vi "Actor Template-Core_Process.vi"(0 "FTW Actor Instance Configuration":string="{\n  \"Identity\": \"ActorName\",\n  \"InboxAddress\": \"inproc://*\",\n  \"LoggerAddress\": \"\",\n  \"My Data\": false,\n  \"Publisher URI\": \"inproc://*\",\n  \"Subscriber URIs\": \"\",\n  \"Refresh Period\": 2\n}", 11 "ErrorIn":errorcluster) -> (15 "Error":errorcluster)   [LabVIEW 2015, in "Actor Template-Core.lvclass"]
uses:
  Actor Template-Core.lvclass
  Actor Template-Core.lvclass/Actor Template-Core.ctl
  source/actor/Instance/FTW-ActorInstance.lvclass/FTW-ActorInstance.ctl
  source/actor/JobSequencer/FTW-SEQ-Current.vi
  source/actor/Message/Base/FTW-Message.lvclass
  source/actor/Connector/FTW-ActorConnector.lvclass
  source/actor/Instance/FTW-ActorInstance.lvclass
  source/actor/Message/Request/FTW-Message-IncomingRequest.lvclass
  source/actor/Publisher/FTW-Publisher.lvclass
  source/actor/Subscriber/FTW-Subscriber.lvclass
panel:
  # "#TODO\nhide controls for a GUI"
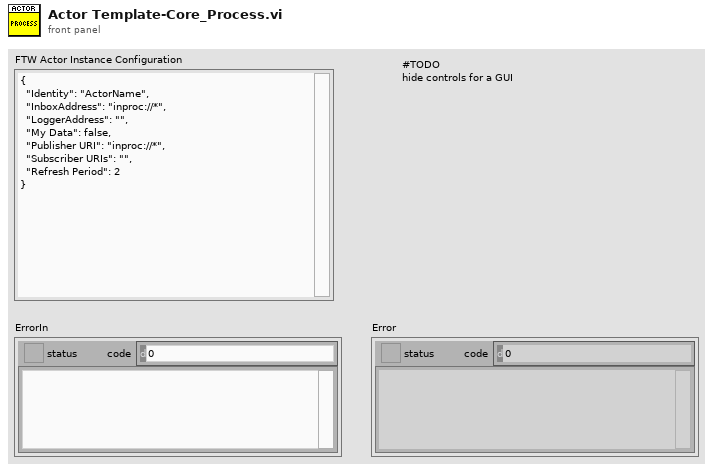
[diagram p1: front panel]
types:
  T1 = cluster{"Incoming Requests":refnum<event-registration>, "Local Messages":refnum<event-registration>, "Subscriber Registration":refnum<event-registration>}
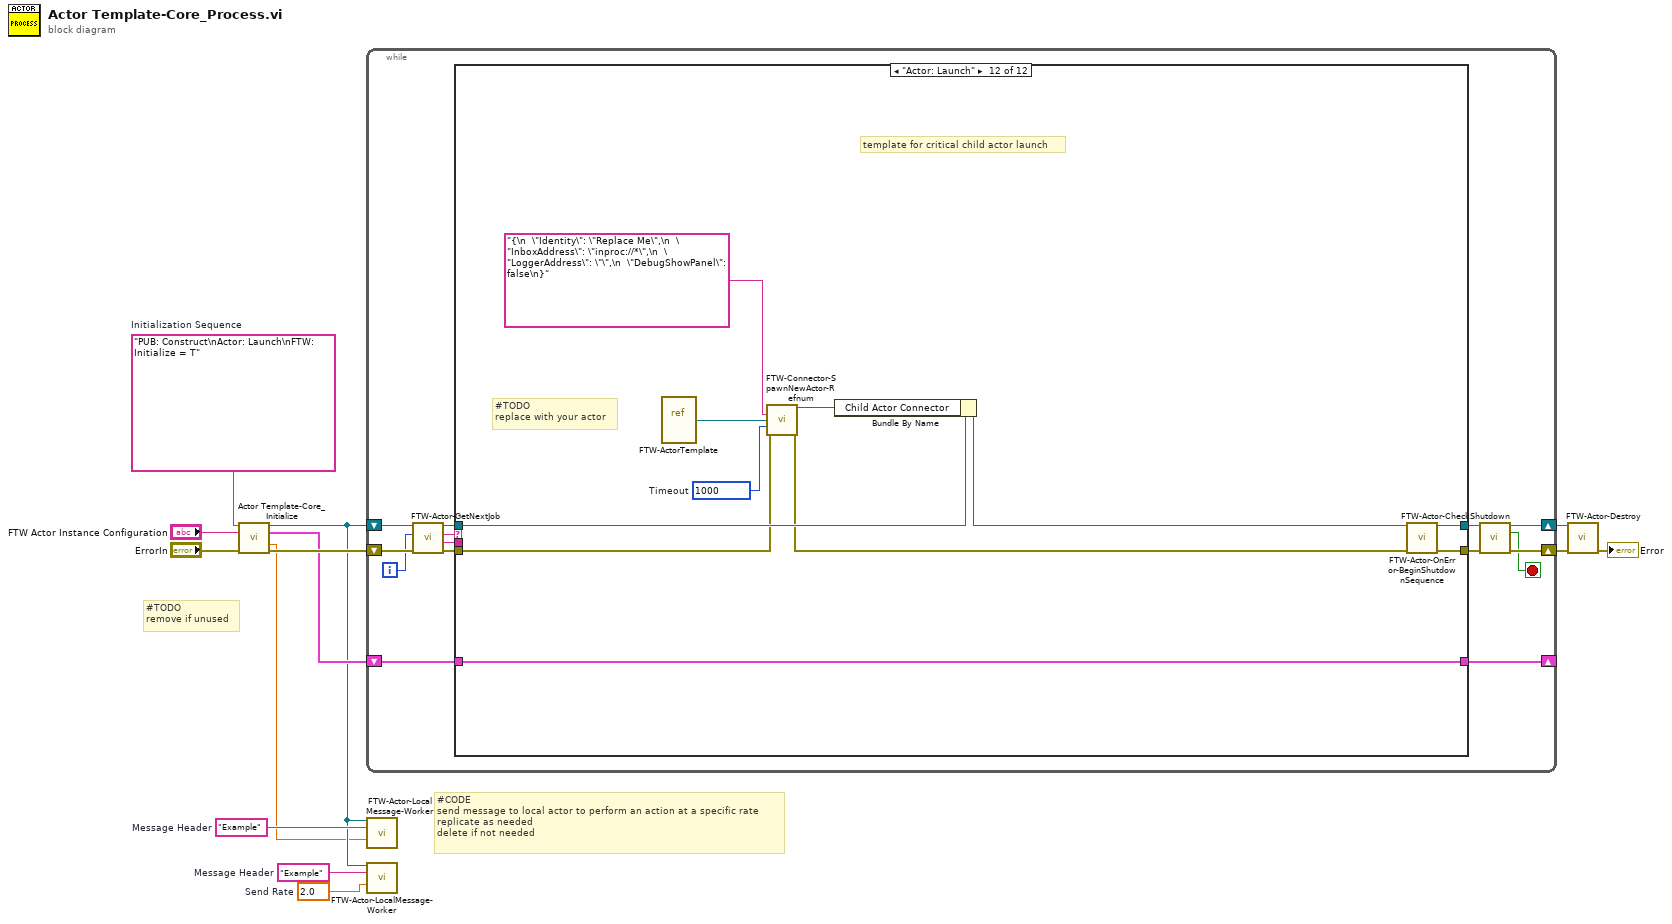
[diagram p0: block diagram]
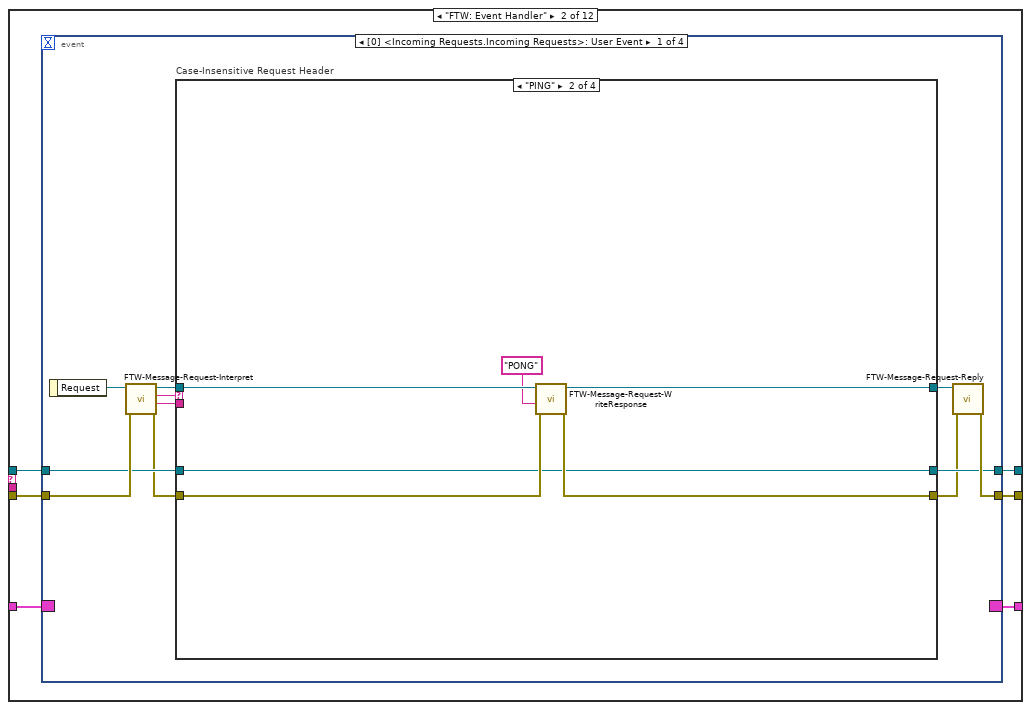
[diagram p3: hidden frame]
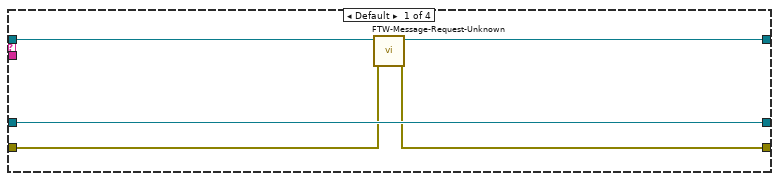
[diagram p4: hidden frame]
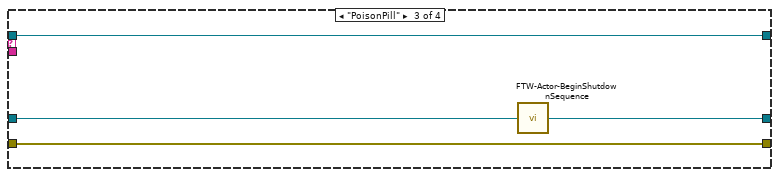
[diagram p5: hidden frame]
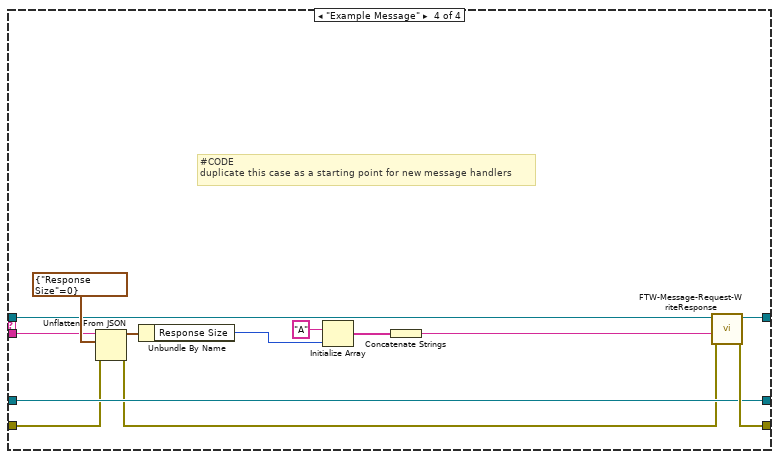
[diagram p6: hidden frame]
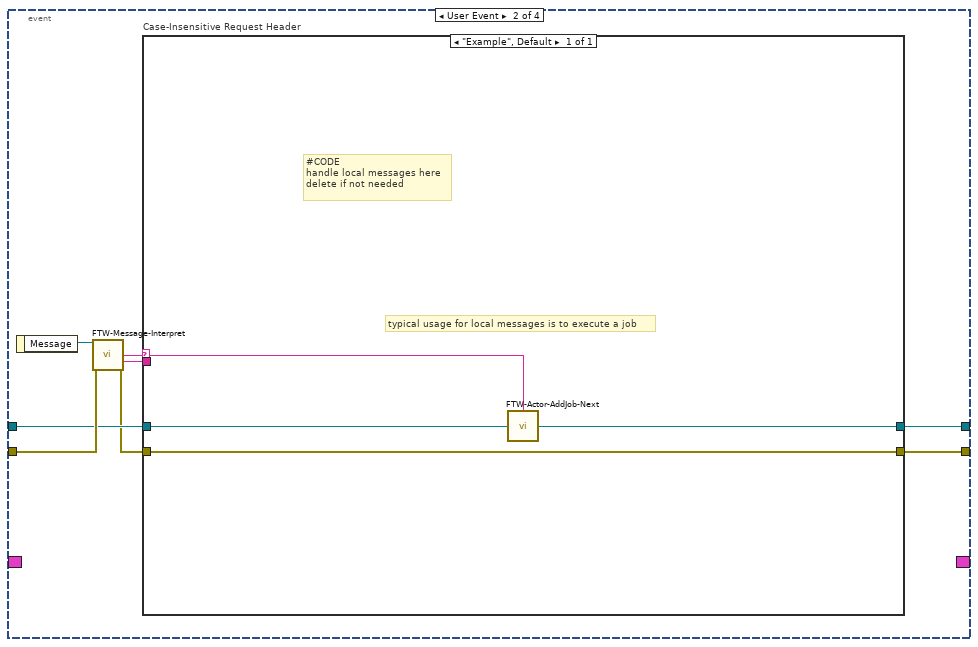
[diagram p7: hidden frame]
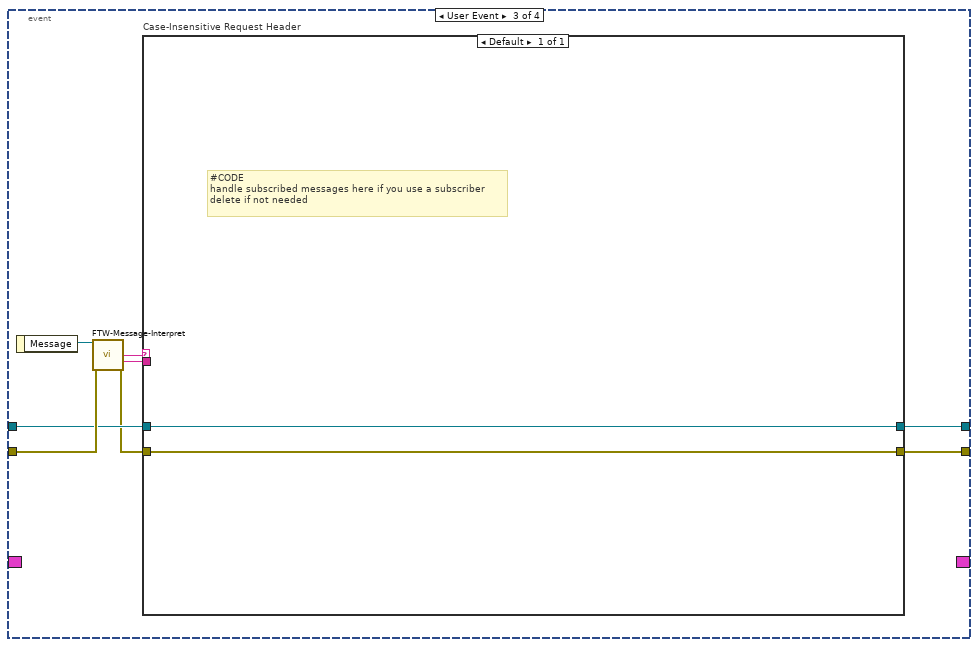
[diagram p8: hidden frame]
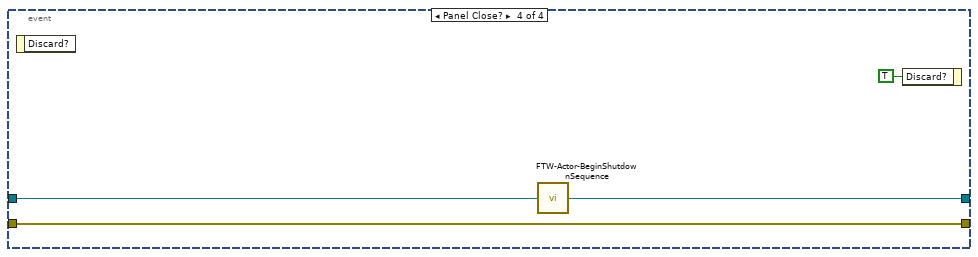
[diagram p9: hidden frame]
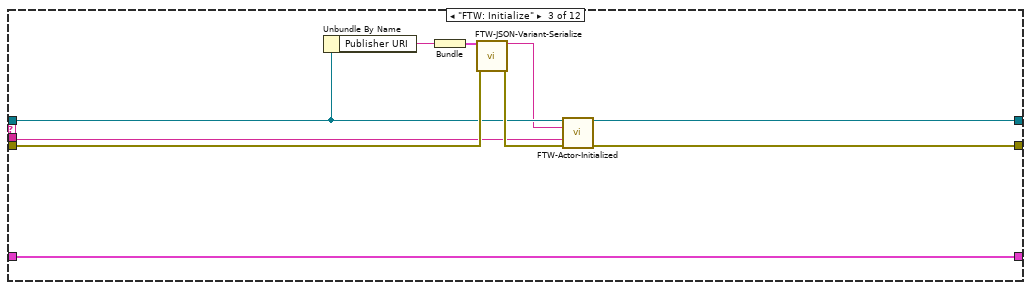
[diagram p10: hidden frame]
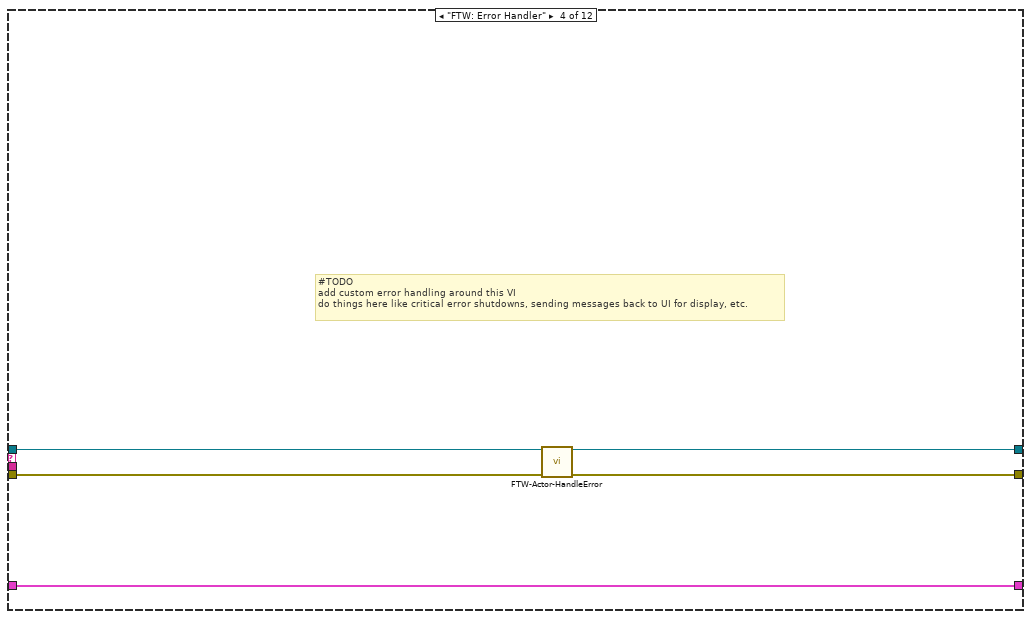
[diagram p11: hidden frame]
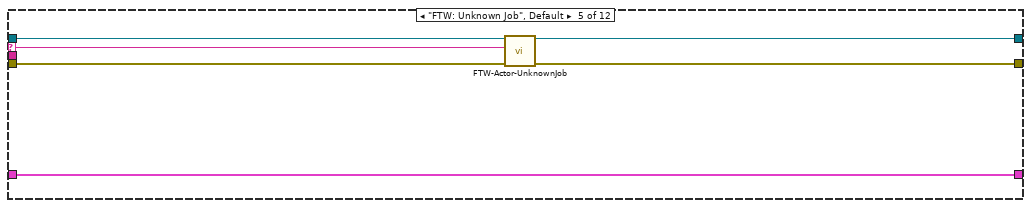
[diagram p12: hidden frame]
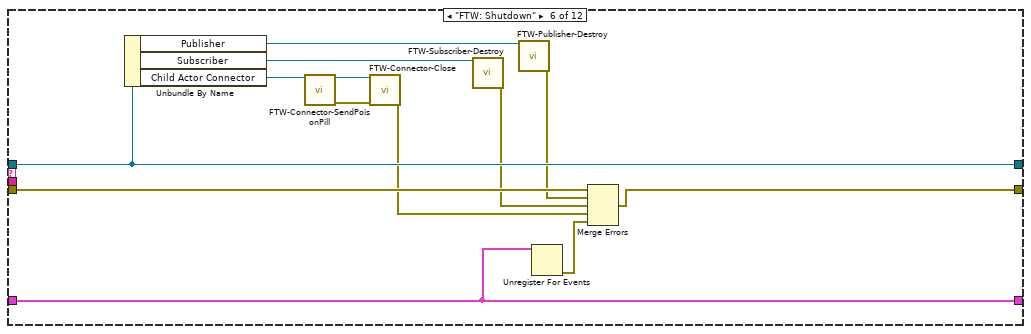
[diagram p13: hidden frame]
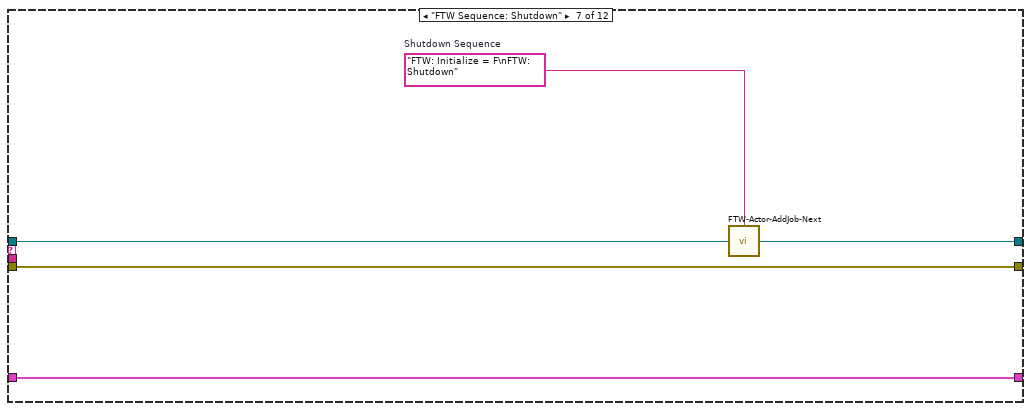
[diagram p14: hidden frame]
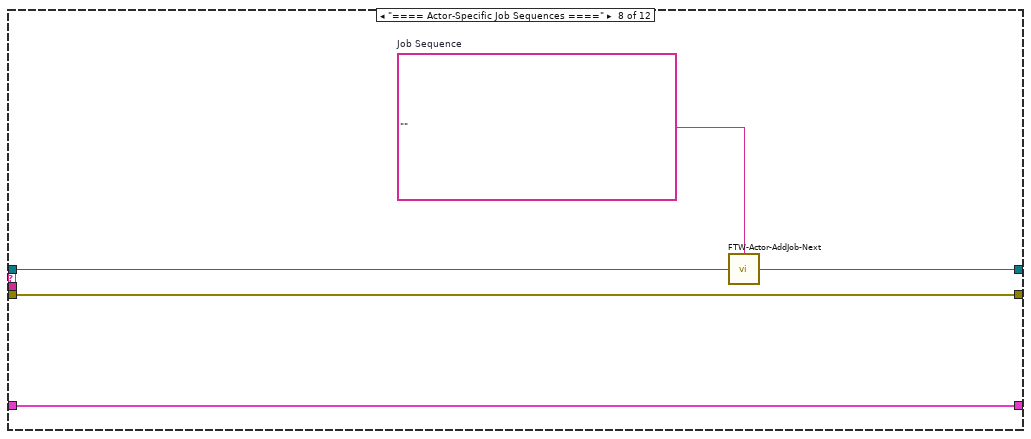
[diagram p15: hidden frame]
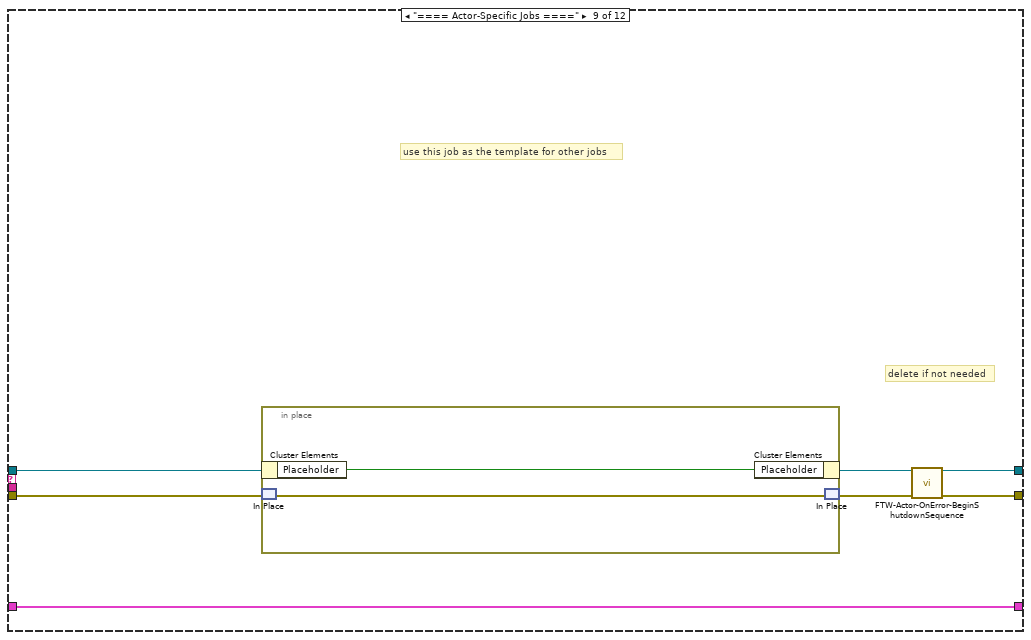
[diagram p16: hidden frame]
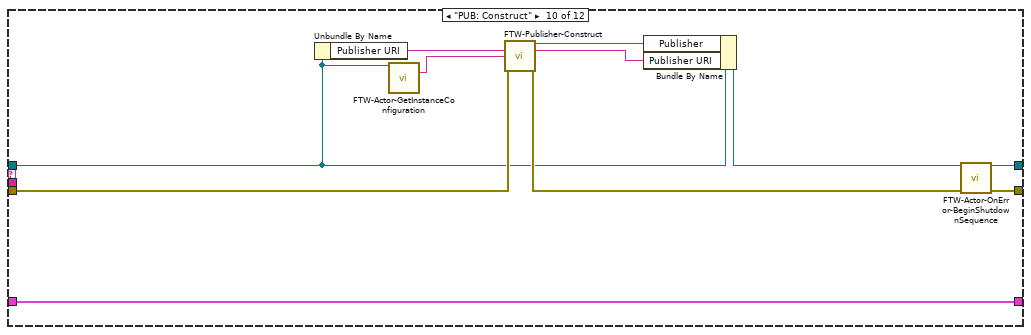
[diagram p17: hidden frame]
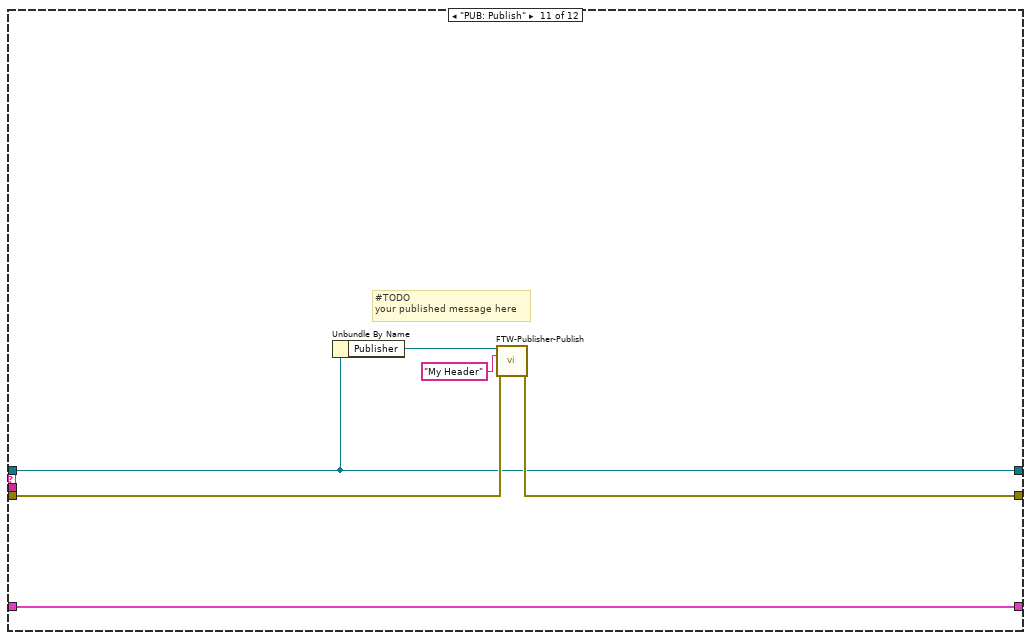
[diagram p18: hidden frame]
diagram:
  w4 = 2.0  # Send Rate
  w3 = "Example"  # Message Header
  w5 = "Example"  # Message Header
  w9 = "PUB: Construct\nActor: Launch\nFTW: Initialize = T"  # Initialization Sequence
  # "#CODE\nsend message to local actor to perform an action at a specific rate\nreplicate as needed\ndelete if not needed"
  # "#TODO\nremove if unused"
  n1 = call "Actor Template-Core_Initialize.vi"("Initialization Sequence"=w9, "FTW Actor Instance Configuration"="FTW Actor Instance Configuration", "error in (no error)"="ErrorIn") -> ("Actor Template-Core out"=w2:refnum<class "Actor Template-Core.lvclass">, "Event Refnums"=w6:T1, "Refresh Period"=w1:dbl, "error out"=w10:errorcluster)  [unwired: 9 in]
  n2 = while {
    shift-right: [w17] -> w12
    shift-left: w10 -> [w24]
    shift-right: [w14] -> _
    shift-left: w6 -> [w27]
    shift-right: [w19] -> w13
    shift-left: w2 -> [w26]
    i -> [w15]
    stop <- w16 stop-if-true
    n3 = call "FTW-Actor-GetNextJob.vi"("error in"=w24, "Jobs Performed"=w15, "FTW Actor Instance"=w26) -> ("error out"=w23:errorcluster, "Job Data"=w21:string, "Job Name"=w22:string, "FTW Actor Instance out"=w25:refnum<class "Actor Template-Core.lvclass">)  [unwired: 5 in]
    n4 = case shown="\"Actor: Launch\"" w22 {
      selector: w22 -> [_ _ _ _ w117 _ _ _ _ _ _ _]
      tunnel: [w29 w36 w107 w112 w120 w134 w139 w144 w148 w161 w169 w181] -> w18
      tunnel: w23 -> [w29 w35 w111 w114 w121 w135 w139 w144 w151 w163 w170 w175]
      tunnel: w27 -> [w30 w31 w109 w116 w122 w132 w140 w145 w152 w165 w171 w182]
      tunnel: [w30 w34 w109 w116 w122 w132 w140 w145 w152 w165 w171 w182] -> w14
      tunnel: w21 -> [_ _ w104 _ _ _ _ _ _ _ _ _]
      tunnel: [w28 w33 w108 w113 w118 w131 w137 w142 w146 w159 w168 w180] -> w20
      tunnel: w25 -> [w28 w32 w106 w115 w119 w131 w138 w143 w149 w156 w168 w179]
      frame "==== Featherweight Framework Jobs ====" {
      }
      frame "FTW: Event Handler" {
        n5 = event shown="[0] <Incoming Requests.Incoming Requests>: User Event" {
          selector: w31 -> [_ _ _ _]
          dyn-events: [_ _ _ _] -> w34
          timeout: _ -> [_ _ _ _]
          tunnel: [w46 w78 w90 w100] -> w36
          tunnel: w35 -> [w45 w82 w94 w100]
          tunnel: [w40 w79 w91 w98] -> w33
          tunnel: w32 -> [w44 w81 w93 w99]
          event User Event {
            n6 = event-data() -> ("Request"=w47:refnum<class "FTW-Message-IncomingRequest.lvclass">)  [unwired: 1 in]
            n7 = call "FTW-Message-Request-Interpret.vi"("error in"=w45, "FTW Incoming Request"=w47) -> ("error out"=w43:errorcluster, "Request Body"=w37:string, "Request Header"=w41:string, "FTW Incoming Request out"=w42:refnum<class "FTW-Message-IncomingRequest.lvclass">)  [unwired: 6 in]
            n8 = case "Case-Insensitive Request Header" shown="\"PING\"" w41 {
              tunnel: [w50 w56 w61 w75] -> w39
              tunnel: w43 -> [w51 w57 w61 w64]
              tunnel: [w52 w55 w62 w73] -> w40
              tunnel: w44 -> [w52 w55 w60 w73]
              tunnel: w42 -> [w49 w58 w59 w65]
              tunnel: [w48 w54 w59 w74] -> w38
              tunnel: w37 -> [_ _ _ w63]
              frame Default {
                n9 = call "FTW-Message-Request-Unknown.vi"("error in"=w51, "FTW Incoming Request"=w49) -> ("error out"=w50:errorcluster, "FTW Incoming Request Out"=w48:refnum<class "FTW-Message-IncomingRequest.lvclass">)  [unwired: 8 in]
              }
              frame "PING" {
                n10 = call "FTW-Message-Request-WriteResponse.vi"("error in"=w57, "Response Body"="PONG" ("Response Header"), "FTW Incoming Request"=w58) -> ("error out"=w56:errorcluster, "FTW Incoming Request out"=w54:refnum<class "FTW-Message-IncomingRequest.lvclass">)  [unwired: 7 in]
              }
              frame "PoisonPill" {
                n11 = call "FTW-Actor-BeginShutdownSequence.vi"("FTW Actor Instance"=w60) -> ("FTW Actor Instance out"=w62:refnum<class "Actor Template-Core.lvclass">)  [unwired: 3 in]
              }
              frame "Example Message" {
                # "#CODE\nduplicate this case as a starting point for new message handlers"
                n12 = Unflatten From JSON(JSON string=w63, type and defaults=cluster{"Response Size":i32} {"Response Size"=0}, error in (no error)=w64) -> (value=w70:cluster{"Response Size":i32}, error out=w72:errorcluster)  [unwired: 4 in]
                n13 = Unbundle By Name(w70) -> ("Response Size"=w69:i32)
                n14 = Initialize Array("A", w69) -> (w67:string[])
                n15 = Concatenate Strings(w67) -> (w66:string)
                n16 = call "FTW-Message-Request-WriteResponse.vi"("error in"=w72, "Response Body"=w66, "FTW Incoming Request"=w65) -> ("error out"=w75:errorcluster, "FTW Incoming Request out"=w74:refnum<class "FTW-Message-IncomingRequest.lvclass">)  [unwired: 7 in]
              }
            }
            n17 = call "FTW-Message-Request-Reply.vi"("FTW: Reply Error"=w39, "FTW Incoming Request"=w38) -> ("error out"=w46:errorcluster)  [unwired: 8 in, 1 out]
          }
          event User Event {
            n18 = event-data() -> ("Message"=w83:refnum<class "FTW-Message.lvclass">)  [unwired: 1 in]
            n19 = call-dynamic "FTW-Message-Interpret.vi"("FTW Message"=w83, "error in"=w82) -> ("Message Header"=w77:string, "Message Body"=w76:string, "error out"=w80:errorcluster)  [unwired: 9 in, 2 out]
            n20 = case "Case-Insensitive Request Header" shown="\"Example\", Default" w77 {
              selector: w77 -> [w84]
              tunnel: [w86] -> w78
              tunnel: w80 -> [w86]
              tunnel: [w85] -> w79
              tunnel: w81 -> [w87]
              tunnel: w76 -> [_]
              frame "Example", Default {
                # "#CODE\nhandle local messages here\ndelete if not needed"
                # "typical usage for local messages is to execute a job"
                n21 = call "FTW-Actor-AddJob-Next.vi"("Add Next in Job Queue"=w84, "FTW Actor Instance"=w87) -> ("FTW Actor Instance out"=w85:refnum<class "Actor Template-Core.lvclass">)  [unwired: 2 in]
              }
            }
          }
          event User Event {
            n22 = event-data() -> ("Message"=w95:refnum<class "FTW-Message.lvclass">)  [unwired: 1 in]
            n23 = call-dynamic "FTW-Message-Interpret.vi"("FTW Message"=w95, "error in"=w94) -> ("Message Header"=w89:string, "Message Body"=w88:string, "error out"=w92:errorcluster)  [unwired: 9 in, 2 out]
            n24 = case "Case-Insensitive Request Header" shown="Default" w89 {
              tunnel: [w96] -> w90
              tunnel: w92 -> [w96]
              tunnel: [w97] -> w91
              tunnel: w93 -> [w97]
              tunnel: w88 -> [_]
              frame Default {
                # "#CODE\nhandle subscribed messages here if you use a subscriber\ndelete if not needed"
              }
            }
          }
          event Panel Close? {
            n25 = event-data() -> ()  [unwired: 1 in, 1 out]
            n26 = call "FTW-Actor-BeginShutdownSequence.vi"("FTW Actor Instance"=w99) -> ("FTW Actor Instance out"=w98:refnum<class "Actor Template-Core.lvclass">)  [unwired: 3 in]
            n27 = event-data("Discard?"=TRUE) -> ()  [unwired: 1 in, 1 out]
          }
        }
      }
      frame "FTW: Initialize" {
        n28 = Unbundle By Name(w106) -> ("Publisher URI"=w105:string)
        n29 = Bundle("Publisher URI"=w105) -> (w103:cluster{"Publisher URI":string})  [unwired: 1 in]
        n30 = call "FTW-JSON-Variant-Serialize.vi"("Variant"=w103, "error in"=w111) -> ("JSON String"=w102:string, "error out"=w110:errorcluster)  [unwired: 12 in]
        n31 = call-dynamic "FTW-Actor-Initialized.vi"("FTW Actor Instance"=w106, "Initialized Response"=w102, "Positive Init?"=w104, "error in"=w110) -> ("FTW Actor Instance out"=w108:refnum<class "Actor Template-Core.lvclass">, "error out"=w107:errorcluster)  [unwired: 10 in]
      }
      frame "FTW: Error Handler" {
        # "#TODO\nadd custom error handling around this VI\ndo things here like critical error shutdowns, sending messages back to UI for display, etc."
        n32 = call-dynamic "FTW-Actor-HandleError.vi"("FTW Actor Instance"=w115, "error in"=w114) -> ("FTW Actor Instance out"=w113:refnum<class "Actor Template-Core.lvclass">, "error out"=w112:errorcluster)  [unwired: 10 in, 2 out]
      }
      frame "FTW: Unknown Job", Default {
        n33 = call-dynamic "FTW-Actor-UnknownJob.vi"("FTW Actor Instance"=w119, "Unknown Job"=w117, "error in"=w121) -> ("FTW Actor Instance out"=w118:refnum<class "Actor Template-Core.lvclass">, "error out"=w120:errorcluster)  [unwired: 11 in]
      }
      frame "FTW: Shutdown" {
        n34 = Unbundle By Name(w131) -> ("Publisher"=w130:refnum<class "FTW-Publisher.lvclass">, "Subscriber"=w128:refnum<class "FTW-Subscriber.lvclass">, "Child Actor Connector"=w126:refnum<class "FTW-ActorConnector.lvclass">)
        n35 = call-dynamic "FTW-Connector-SendPoisonPill.vi"("FTW Actor Connector"=w126) -> ("FTW Actor Connector out"=w125:refnum<class "FTW-ActorConnector.lvclass">, "error out"=w124:errorcluster)  [unwired: 9 in, 4 out]
        n36 = call-dynamic "FTW-Connector-Close.vi"("FTW Actor Connector"=w125, "error in"=w124) -> ("error out"=w123:errorcluster)  [unwired: 13 in]
        n37 = call "FTW-Subscriber-Destroy.vi"("FTW-Subscription In"=w128) -> ("error out"=w127:errorcluster)  [unwired: 14 in]
        n38 = call "FTW-Publisher-Destroy.vi"("FTW-Publisher In"=w130) -> ("error out"=w129:errorcluster)  [unwired: 14 in]
        n39 = Unregister For Events(event registration refnum=w132) -> (error out=w133:errorcluster)  [unwired: 1 in]
        n40 = Merge Errors(w135, w129, w127, w123, w133) -> (w134:errorcluster)
      }
      frame "FTW Sequence: Shutdown" {
        w136 = "FTW: Initialize = F\nFTW: Shutdown"  # Shutdown Sequence
        n41 = call "FTW-Actor-AddJob-Next.vi"("Add Next in Job Queue"=w136, "FTW Actor Instance"=w138) -> ("FTW Actor Instance out"=w137:refnum<class "Actor Template-Core.lvclass">)  [unwired: 2 in]
      }
      frame "==== Actor-Specific Job Sequences ====" {
        w141 = ""  # Job Sequence
        n42 = call "FTW-Actor-AddJob-Next.vi"("Add Next in Job Queue"=w141, "FTW Actor Instance"=w143) -> ("FTW Actor Instance out"=w142:refnum<class "Actor Template-Core.lvclass">)  [unwired: 2 in]
      }
      frame "==== Actor-Specific Jobs ====" {
        # "delete if not needed"
        # "use this job as the template for other jobs"
        n43 = in-place {
          n44 = in-place-cluster #1(w149) -> ("Placeholder"=w153:bool)
          n45 = in-place-match #2(w151) -> (w154:errorcluster)
          n46 = in-place-cluster #1("Placeholder"=w153) -> (w147:refnum<class "Actor Template-Core.lvclass">)
          n47 = in-place-match #2(w154) -> (w150:errorcluster)
        }
        n48 = call-dynamic "FTW-Actor-OnError-BeginShutdownSequence.vi"("FTW Actor Instance"=w147, "error in"=w150) -> ("FTW Actor Instance out"=w146:refnum<class "Actor Template-Core.lvclass">, "error out"=w148:errorcluster)  [unwired: 12 in]
      }
      frame "PUB: Construct" {
        n49 = Unbundle By Name(w156) -> ("Publisher URI"=w157:string)
        n50 = call "FTW-Actor-GetInstanceConfiguration.vi"("FTW Actor Instance"=w156) -> ("Identity"=w155:string)  [unwired: 12 in, 2 out]
        n51 = call "FTW-Publisher-Construct.vi"("Address"=w157, "Identity"=w155, "error in"=w163) -> ("FTW-Publisher Out"=w164:refnum<class "FTW-Publisher.lvclass">, "Actual Address"=w158:string, "error out"=w162:errorcluster)  [unwired: 10 in]
        n52 = Bundle By Name(cluster=w156, "Publisher"=w164, "Publisher URI"=w158) -> (w160:refnum<class "Actor Template-Core.lvclass">)
        n53 = call-dynamic "FTW-Actor-OnError-BeginShutdownSequence.vi"("FTW Actor Instance"=w160, "error in"=w162) -> ("FTW Actor Instance out"=w159:refnum<class "Actor Template-Core.lvclass">, "error out"=w161:errorcluster)  [unwired: 12 in]
      }
      frame "PUB: Publish" {
        # "#TODO\nyour published message here"
        n54 = Unbundle By Name(w168) -> ("Publisher"=w167:refnum<class "FTW-Publisher.lvclass">)
        n55 = call "FTW-Publisher-Publish.vi"("FTW-Publisher In"=w167, "Header"="My Header", "error in"=w170) -> ("error out"=w169:errorcluster)  [unwired: 11 in, 1 out]
      }
      frame "Actor: Launch" {
        w178 = 1000  # Timeout
        # "#TODO\nreplace with your actor"
        # "template for critical child actor launch"
        n56 = vi-ref "FTW-ActorTemplate.vi"() -> (w177:refnum<vi>)
        n57 = call "FTW-Connector-SpawnNewActor-Refnum.vi"("Configuration"="{\n  \"Identity\": \"Replace Me\",\n  \"InboxAddress\": \"inproc://*\",\n  \"LoggerAddress\": \"\",\n  \"DebugShowPanel\": false\n}", "Actor VI Refnum"=w177, "Timeout"=w178, "error in"=w175) -> ("FTW Actor Connector"=w172:refnum<class "FTW-ActorConnector.lvclass">, "error out"=w174:errorcluster)  [unwired: 8 in, 2 out]
        n58 = Bundle By Name(cluster=w179, "Child Actor Connector"=w172) -> (w173:refnum<class "Actor Template-Core.lvclass">)
        n59 = call-dynamic "FTW-Actor-OnError-BeginShutdownSequence.vi"("FTW Actor Instance"=w173, "error in"=w174) -> ("FTW Actor Instance out"=w180:refnum<class "Actor Template-Core.lvclass">, "error out"=w181:errorcluster)  [unwired: 12 in]
      }
    }
    n60 = call "FTW-Actor-CheckShutdown.vi"("FTW Actor Instance"=w20, "error in"=w18) -> ("FTW Actor Instance out"=w19:refnum<class "Actor Template-Core.lvclass">, "Shutdown?"=w16:bool, "error out"=w17:errorcluster)  [unwired: 11 in]
  }
  n61 = call-dynamic "FTW-Actor-LocalMessage-Worker.vi"("FTW-ActorInstance In"=w2, "Message Header"=w5, "Send Rate"=w1) -> ()  [unwired: 13 in]
  n62 = call-dynamic "FTW-Actor-LocalMessage-Worker.vi"("FTW-ActorInstance In"=w2, "Message Header"=w3, "Send Rate"=w4) -> ()  [unwired: 13 in]
  n63 = call-dynamic "FTW-Actor-Destroy.vi"("FTW Actor Instance"=w13, "error in"=w12) -> ("error out"=→"Error":errorcluster)  [unwired: 13 in]
